vi "Audio_Transformation_Setted_Frequency_v002.vi"() -> ()   [LabVIEW 2019]
uses:
  <vilib>/sound2/lvsound2.llb/Sound Data Format.ctl
  <vilib>/sound2/lvsound2.llb/Sound Input Read (DBL).vi
  <vilib>/addons/Time Frequency Analysis/Transform.llb/TFA Online Gabor Transform (Real).vi
  <vilib>/addons/_Advanced Signal Processing/NI_AdvSigProcTFA.lvlib
panel:
  out "Noise Speech":dbl[](graph)
  out "u(t)":dbl(graph)
  out "V(t)":dbl(graph)
  in  "Address selector":i32[](array[numeric])
  in  "Neuron Type":T1(ring)
  out "max index(es)":i32
  out "max value":dbl
  out "Waveform Graph":dbl[](graph)
  out "Magnitude of Gabor Coefficients":dbl[][](graph)
  in  "Stop":bool
  # "Step two : Graph of the amplitude of the Gabor coefficient of the different bins"
  # "Step three : Spike Response of the neuron"
  # "Step one: Sound recorded from the computer"
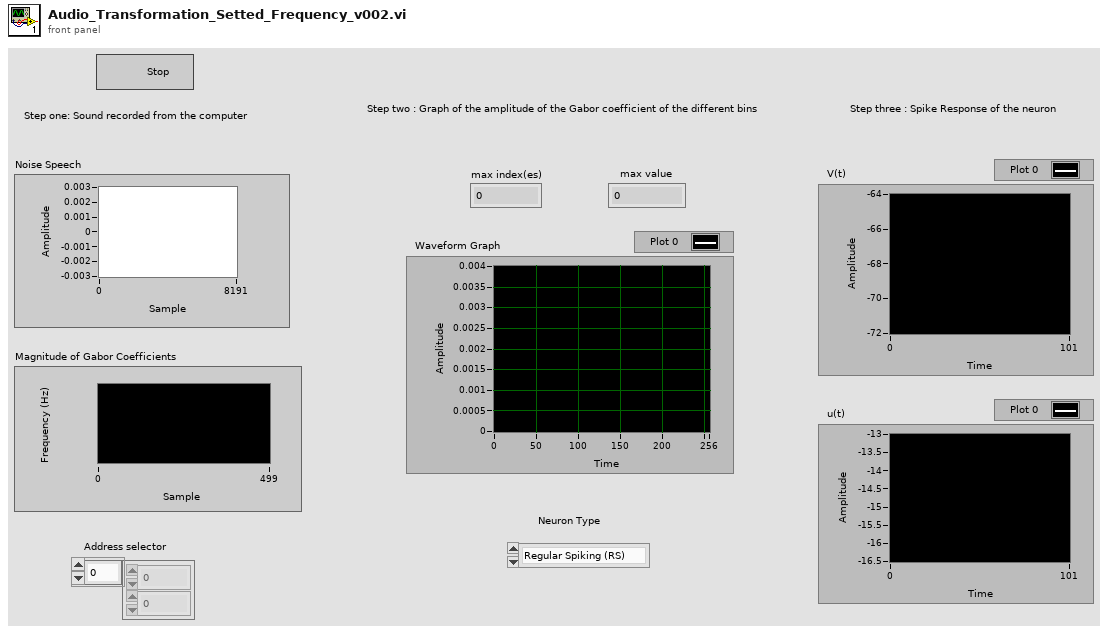
[diagram p1: front panel]
types:
  T1 = enum16{"Regular Spiking (RS)", "Intrinsically Bursting (IB)", "Chattering (CH)", "Fast Spiking (FS)", "Thalamo-Cortical 1 (TC1)", "Thalamo-Cortical 2 (TC2)", "Resonator (RZ)", "Low-Threshold Spiking (LTS)", "Phasic Spiking (PS)"}
  T2 = typedef "Sound Data Format.ctl" = cluster{"sample rate (S/s)":dbl, "number of channels":i32, "bits per sample":i32}
  T3 = typedef "Sound Input Task ID.ctl" = u32
  T4 = cluster{"analysis window":dbl[], "dM (time steps)":i32, "N (frequency bins)":i32}
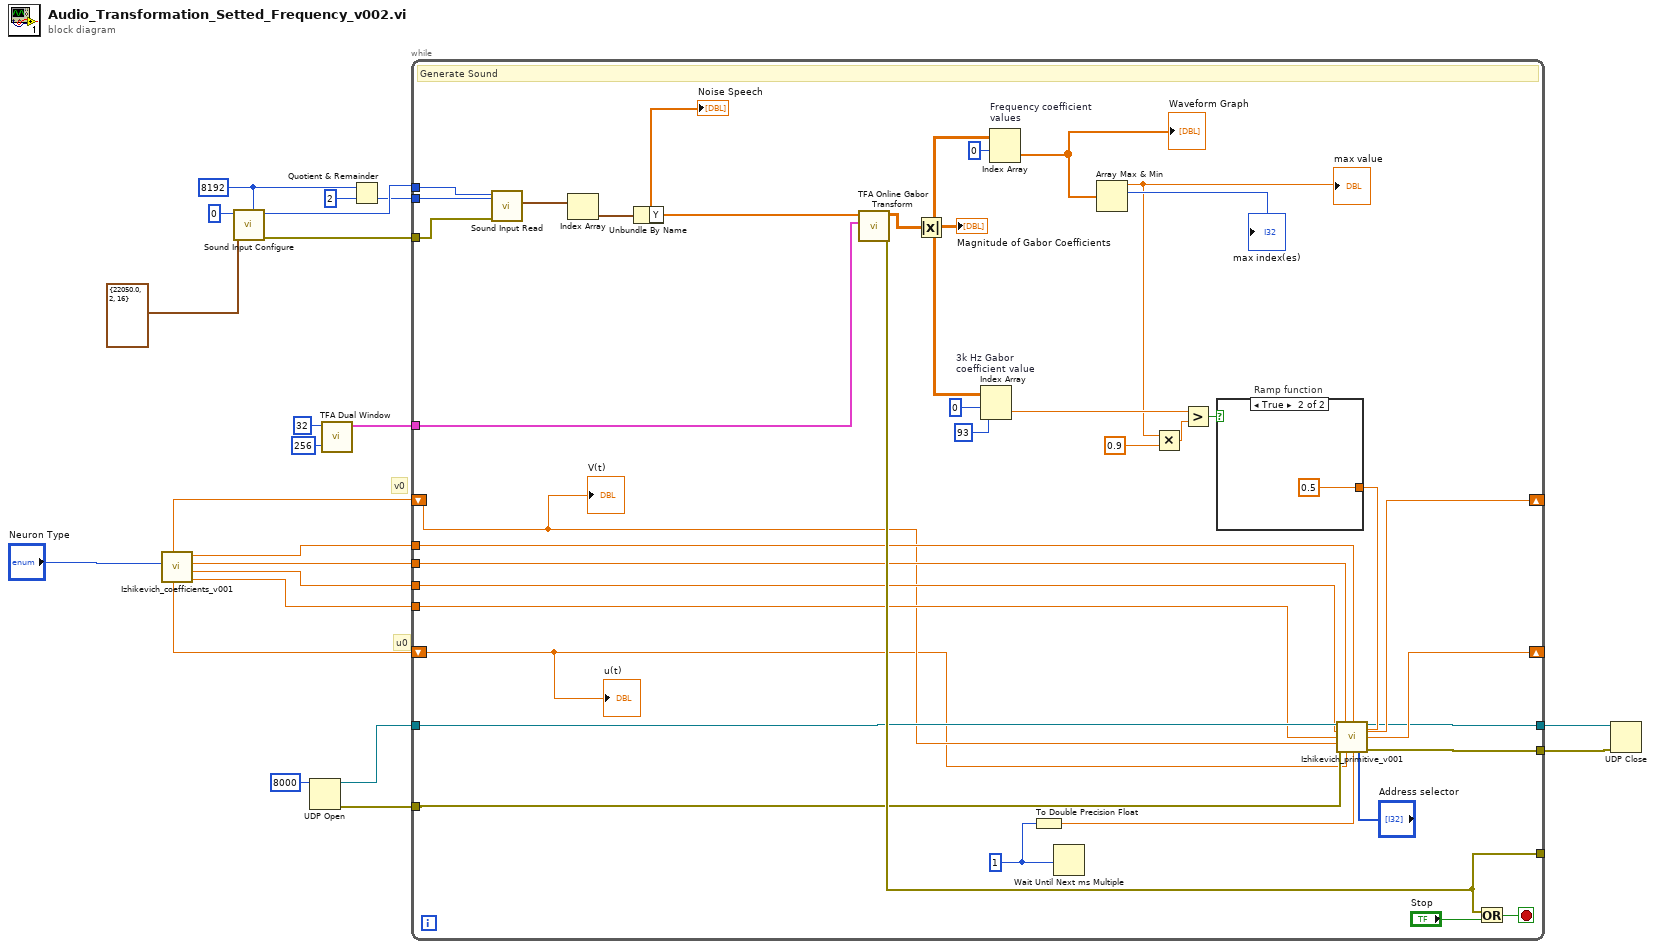
[diagram p0: block diagram]
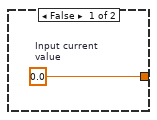
[diagram p2: hidden frame]
diagram:
  w5 = 8192 ("number of samples/ch")
  # "u0"
  # "v0"
  n1 = call "Izhikevich_coefficients_v001.vi"("Neuron Type"="Neuron Type") -> ("d"=w13:dbl, "c"=w14:dbl, "b"=w15:dbl, "a"=w16:dbl, "u0"=w17:dbl, "v0"=w18:dbl)  [unwired: 3 in]
  n2 = call <vilib>:"Sound Input Configure.vi"("number of samples/ch"=w5, "sound format"=T2 {"sample rate (S/s)"=22050.0, "number of channels"=2, "bits per sample"=16}, "device ID"=u32 0) -> ("error out"=w2:errorcluster, "task ID"=w3:T3)  [unwired: 7 in]
  n3 = UDP Open(11:u16 8000 ("port")) -> (port=w11:refnum<k16>, 0:w10:errorcluster)  [unwired: 4 in, 1 out]
  n4 = call <vilib>:"TFA Dual Window.vi"("N (frequency bins)"=256, "dM (time steps)"=32) -> ("analysis info"=w20:T4)  [unwired: 7 in, 2 out]
  n5 = Quotient & Remainder(x=w5, y=2) -> (floor(x/y)=w1:i32)  [unwired: 1 out]
  n6 = while {
    tunnel: [w50] -> _
    tunnel: w20 -> [w58]
    shift-right: [w37] -> _
    shift-left: w18 -> [w33]
    shift-right: [w36] -> _
    shift-left: w17 -> [w32]
    tunnel: w16 -> [w46]
    tunnel: w15 -> [w45]
    tunnel: w14 -> [w43]
    tunnel: w13 -> [w42]
    tunnel: w11 -> [w44]
    tunnel: w10 -> [w41]
    tunnel: [w35] -> w9
    tunnel: [w34] -> w8
    tunnel: w3 -> [w30]
    tunnel: w2 -> [w29]
    tunnel: w1 -> [w31]
    stop <- w59 stop-if-true
    w39 = u32 1 ("millisecond multiple")
    # "Generate Sound"
    n7 = call-poly <vilib>:"Sound Input Read.vi"("number of samples/ch"=w31, "error in (no error)"=w29, "task ID"=w30) -> ("data"=w27:waveform(dbl)[])  [unwired: 6 in, 2 out]
    n8 = Index Array(array=w27) -> (element=w28:waveform(dbl))  [unwired: 1 in]
    n9 = Unbundle By Name(w28) -> ("Y"=w26:dbl[])
    "Noise Speech" <- w26
    n10 = call-poly <vilib>:"TFA Online Gabor Transform.vi"("transform info"=w58, "signal"=w26) -> ("error out"=w50:errorcluster, "Gabor coef"=w57:cdb[][])  [unwired: 7 in, 1 out]
    n11 = Absolute Value(x=w57) -> (abs(x)=w53:dbl[][])
    "Magnitude of Gabor Coefficients" <- w53
    n12 = Index Array "3k Hz Gabor \ncoefficient value"(array=w53, index (row)=0, index (col)=93 ("disabled index (col)")) -> (element=w49:dbl)
    n13 = Index Array "Frequency coefficient \nvalues"(array=w53, index (row)=0) -> (element=w55:dbl[])  [unwired: 1 in]
    "Waveform Graph" <- w55
    n14 = To Double Precision Float(number=w39) -> (double precision float=w38:dbl)
    n15 = Wait Until Next ms Multiple(millisecond multiple=w39) -> ()  [unwired: 1 out]
    n16 = Array Max & Min(array=w55) -> (max value=w23:dbl, max index (indices)=→"max index(es)":i32)  [unwired: 2 out]
    "max value" <- w23
    n17 = Multiply(x=w23, y=0.9) -> (x*y=w25:dbl)
    n18 = Greater?(x=w49, y=w25) -> (0:w48:bool)
    n19 = case "Ramp function" shown="True" w48 {
      tunnel: [w61 0.5 ("Input current \nvalue")] -> w47
      frame False {
        w61 = 0.0  # Input current  value
      }
      frame True {
      }
    }
    n20 = call "Izhikevich_primitive_v001.vi"("UDP Network Connection in"=w44, "b"=w45, "a"=w46, "I"=w47, "c"=w43, "d"=w42, "v(t)"=w33, "error in (no error)"=w41, "u(t)"=w32, "Numeric"=w38, "Address selector"="Address selector") -> ("UDP Network Connection out"=w34:refnum<k16>, "v(t+dt)"=w37:dbl, "u(t+dt)"=w36:dbl, "error out"=w35:errorcluster)  [unwired: 1 in]
    n21 = Or(x=w50, y="Stop") -> (x .or. y?=w59:bool)
    "V(t)" <- w33
    "u(t)" <- w32
  }
  n22 = UDP Close(connection ID=w8, 8:w9) -> ()  [unwired: 2 out]
